vi "Write Path.vi"(8 "error in (no error)":errorcluster, 9 "Filename [Configuration.ini]":string="Configuration.ini", 10 "Path":path, 11 "Configuration in":refnum<class "Configuration.lvclass">) -> (0 "error out":errorcluster, 3 "Configuration out":refnum<class "Configuration.lvclass">)   [LabVIEW 2019, in "Configuration.lvclass"]
uses:
  Configuration.lvclass
  Configuration.lvclass/Configuration.ctl
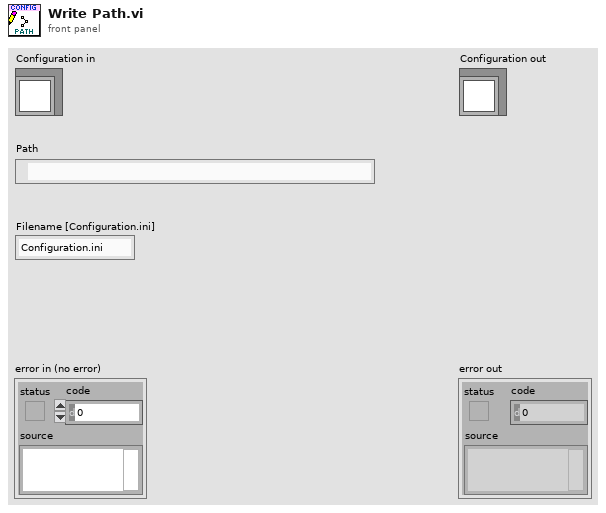
[diagram p1: front panel]
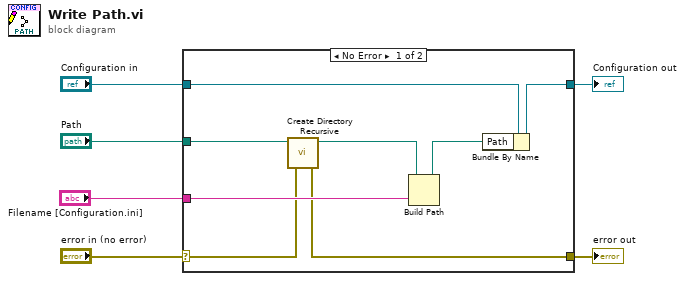
[diagram p0: block diagram]
diagram:
  n1 = case shown="No Error" "error in (no error)" {
    selector: "error in (no error)" -> [w8 w15]
    tunnel: [w7 w15] -> w5
    tunnel: [w13 w16] -> w3
    tunnel: "Configuration in" -> [w14 w16]
    tunnel: "Path" -> [w9 _]
    tunnel: "Filename [Configuration.ini]" -> [w11 _]
    frame No Error {
      n2 = call <vilib>:"Create Directory Recursive.vi"("error in (no error)"=w8, "directory"=w9) -> ("error out"=w7:errorcluster, "directory copy"=w10:path)  [unwired: 3 in, 1 out]
      n3 = Build Path(base path=w10, name or relative path=w11) -> (appended path=w12:path)
      n4 = Bundle By Name(cluster=w14, "Path"=w12) -> (w13:refnum<class "Configuration.lvclass">)
    }
    frame Error {
    }
  }
  "error out" <- w5
  "Configuration out" <- w3
